vi "Maximum Speed 결정 (수정 해야함).vi"(2 "LIDAR magn. (m)":dbl[](array[numeric]), 3 "Max Speed":dbl) -> (1 "Target speed":dbl)   [LabVIEW 2016]
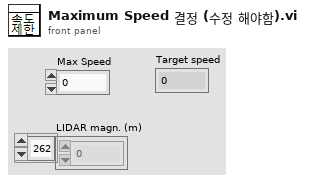
[diagram p1: front panel]
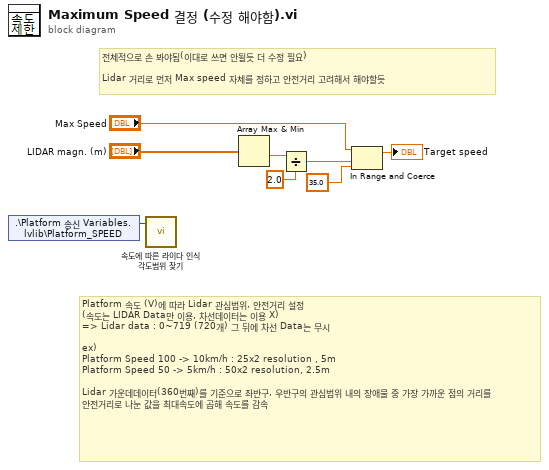
[diagram p0: block diagram]
diagram:
  # "전체적으로 손 봐야됨(이대로 쓰면 안될듯 더 수정 필요)\n\nLidar 거리로 먼저 Max speed 자체를 정하고 안전거리 고려해서 해야할듯"
  # "Platform 속도 (V)에 따라 Lidar 관심범위, 안전거리 설정\n(속도는 LIDAR Data만 이용, 차선데이터는 이용 X) \n=> Lidar data : 0~719 (720개) 그 뒤에 차선 Data는 무시\n\nex)\nPlatform Speed 100 -> 10km/h : 25x2 resolution , 5m\nPlatform Speed 50 -> 5km/h : 50x2 resolution, 2.5m\n\nLidar 가운데데이터(360번째)를 기준으로 좌반구, 우반구의 관심범위 내의 장애물 중 가장 가까운 점의 거리를 안전거리로 나눈 값을 최대속도에 곱해 속도를 감속"
  n1 = shared-variable ".\\Platform 송신 Variables.lvlib\\Platform_SPEED"() -> (w8:u16)  [unwired: 1 in, 1 out]
  n2 = call "속도에 따른 라이다 인식 각도범위 찾기.vi"("speed"=w8) -> ()  [unwired: 1 in, 2 out]
  n3 = Array Max & Min(array="LIDAR magn. (m)") -> (min value=w6:dbl)  [unwired: 3 out]
  n4 = Divide(x=w6, y=2.0) -> (x/y=w4:dbl)
  n5 = In Range and Coerce(upper limit="Max Speed", x=w4, lower limit=35.0 ("하위 리미트")) -> (coerced(x)=→"Target speed":dbl)  [unwired: 1 out]
